vi "Configure Serial.vi"(8 "error in":errorcluster, 10 "Serial Config":T1={"baud rate"=19200, "data bits"=8, "stop bits"=10, "parity"=0, "flow control"=0, "endModeforReads"=2, "endModeforWrites"=2} {"stop bits" items=["1.0"=10, "1.5"=15, "2.0"=20]; "parity" items=["None", "Odd", "Even", "Mark", "Space"]; "flow control" items=["None", "XON/XOFF", "RTS/CTS", "XON/XOFF & RTS/CTS", "DTR/DSR", "XON/XOFF & DTR/DSR"]; "endModeforReads" items=["None", "Last Bit", "TermChar"]; "endModeforWrites" items=["None", "Last Bit", "TermChar", "Break"]}, 11 "Serial Session in":refnum<class "Serial Session.lvclass">) -> (0 "error out":errorcluster, 3 "Serial Session out":refnum<class "Serial Session.lvclass">)   [LabVIEW 2019, in "Serial Session.lvclass"]
uses:
  Serial Session.lvclass
  Typedefs/Serial Config.ctl
  Serial Session.lvclass/Serial Session.ctl
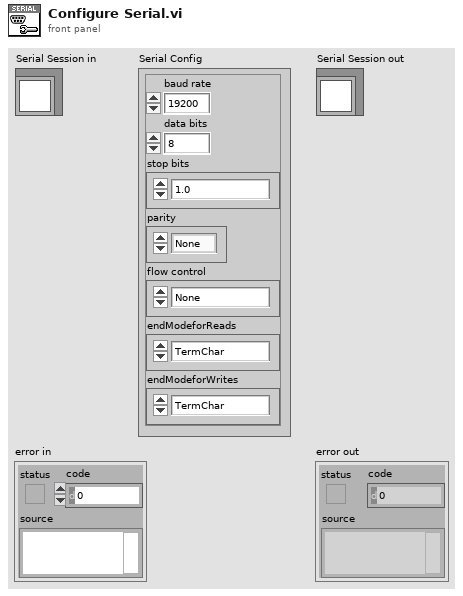
[diagram p1: front panel]
types:
  T1 = typedef "Serial Session.lvclass/Serial Config.ctl" = cluster{"baud rate":u32, "data bits":u16, "stop bits":u16, "parity":u16, "flow control":u16, "endModeforReads":u16, "endModeforWrites":u16}
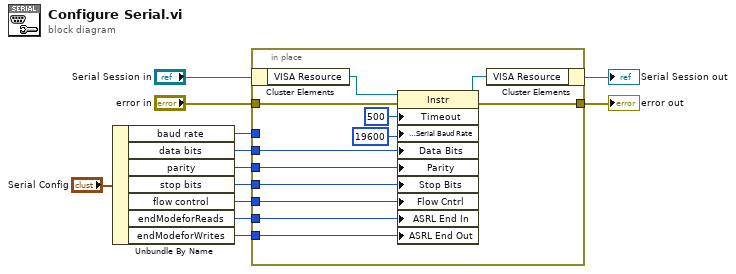
[diagram p0: block diagram]
diagram:
  n1 = Unbundle By Name("Serial Config") -> ("baud rate"=w10:u32, "data bits"=w9:u16, "parity"=w8:u16, "stop bits"=w7:u16, "flow control"=w6:u16, "endModeforReads"=w5:u16, "endModeforWrites"=w4:u16)
  n2 = in-place {
    in-place-border: w10 -> [_]
    in-place-border: w9 -> [w22]
    in-place-border: w8 -> [w21]
    in-place-border: w7 -> [w20]
    in-place-border: w6 -> [w19]
    in-place-border: w5 -> [w18]
    in-place-border: w4 -> [w17]
    in-place-border: "error in" -> [w24]
    in-place-border: [w23] -> w2
    n3 = in-place-cluster #1("Serial Session in") -> ("VISA Resource"=w16:refnum<visa-resource-name>)
    n4 = property class="Instr"(reference=w16, error in=w24, "Timeout"=u32 500 ("General Settings:Timeout Value"), "Serial Settings:Serial Baud Rate"=u32 19600 ("Serial Settings:Baud Rate"), "Data Bits"=w22, "Parity"=w21, "Stop Bits"=w20, "Flow Cntrl"=w19, "ASRL End In"=w18, "ASRL End Out"=w17) -> (reference out=w15:refnum<visa-resource-name>, error out=w23:errorcluster)
    n5 = in-place-cluster #1("VISA Resource"=w15) -> (→"Serial Session out":refnum<class "Serial Session.lvclass">)
  }
  "error out" <- w2
